vi "solar_tcp Core Server.vi"(7 "Action":T4, 8 "error in (no error)":errorcluster, 9 "Read Timeout (0ms)":i32, 10 "Message to Send":string, 11 "TCP Data in":T1 {"Debug"."Time" format="%<%Y-%m-%d\n%H:%M:%S%3u>T"}) -> (0 "error out":errorcluster, 1 "Connected":bool, 2 "Message Read/Sent":string, 3 "TCP Data out":T1 {"Debug"."Time" format="%<%Y-%m-%d\n%H:%M:%S%3u>T"})   [LabVIEW 2018]
doc: "This is the TCP Server core state machine that handles a TCP session. The <b>Message to Send</b> and <b>Message Read</b> should contain the entire TCP message including the header. Before writing the <b>Message to Send</b> the length field is updated as defined by the configuration header length offset and size. The total length field is typically the first 4 bytes of the message which includes the total packet size."
uses:
  solar_tcp_ctl Action.ctl
  solar_tcp_ctl Data.ctl
  solar_tcp_ctl Config.ctl
  solar_tcp_ctl Debug.ctl
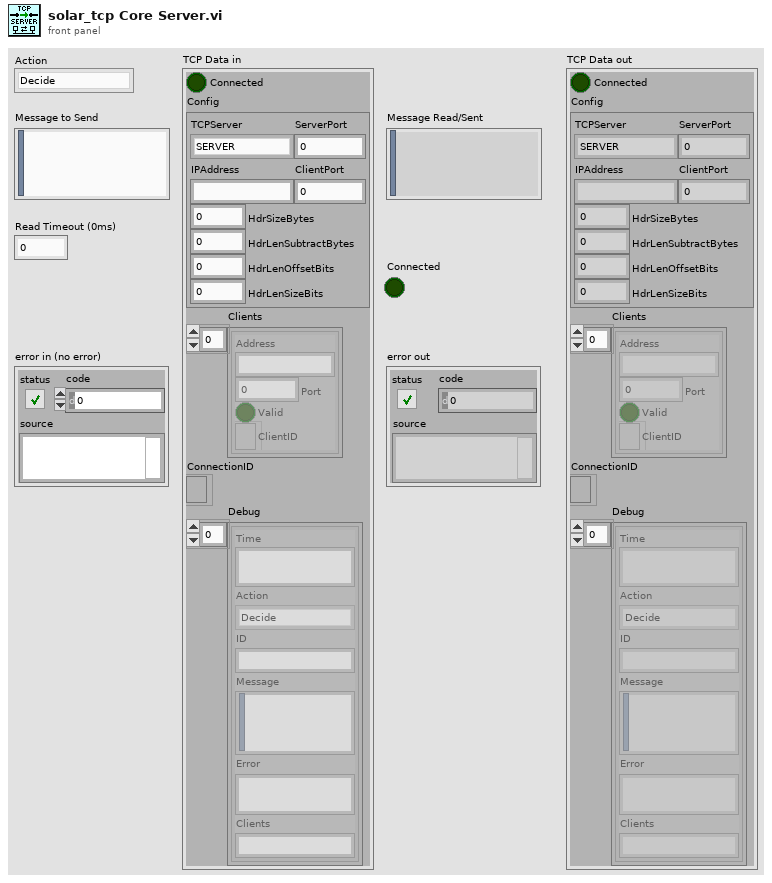
[diagram p1: front panel]
types:
  T1 = typedef "solar_tcp_ctl Data.ctl" = cluster{"Connected":bool, "Config":T2, "Clients":cluster{"Address":string, "Port":u16, "Valid":bool, "ClientID":refnum<k5>}[], "ConnectionID":refnum<k5>, "Debug":T3[]}
  T2 = typedef "solar_tcp_ctl Config.ctl" = cluster{"TCPServer":enum8{"SERVER", "CLIENT"}, "ServerPort":u16, "IPAddress":string, "ClientPort":u16, "HdrSizeBytes":i32, "HdrLenSubtractBytes":i32, "HdrLenOffsetBits":i32, "HdrLenSizeBits":i32}
  T3 = typedef "solar_tcp_ctl Debug.ctl" = cluster{"Time":timestamp, "Action":T4, "ID":string, "Message":string, "Error":string, "Clients":string}
  T4 = typedef "solar_tcp_ctl Action.ctl" = enum16{"Decide", "CreateListener", "Open", "Read", "Write", "Close", "Shutdown", "Done", "ChangePort"}
  T5 = cluster{"Address":string, "Port":u16, "Valid":bool, "ClientID":refnum<k5>}[]
  T6 = cluster{"Address":string, "Port":u16, "Valid":bool, "ClientID":refnum<k5>}
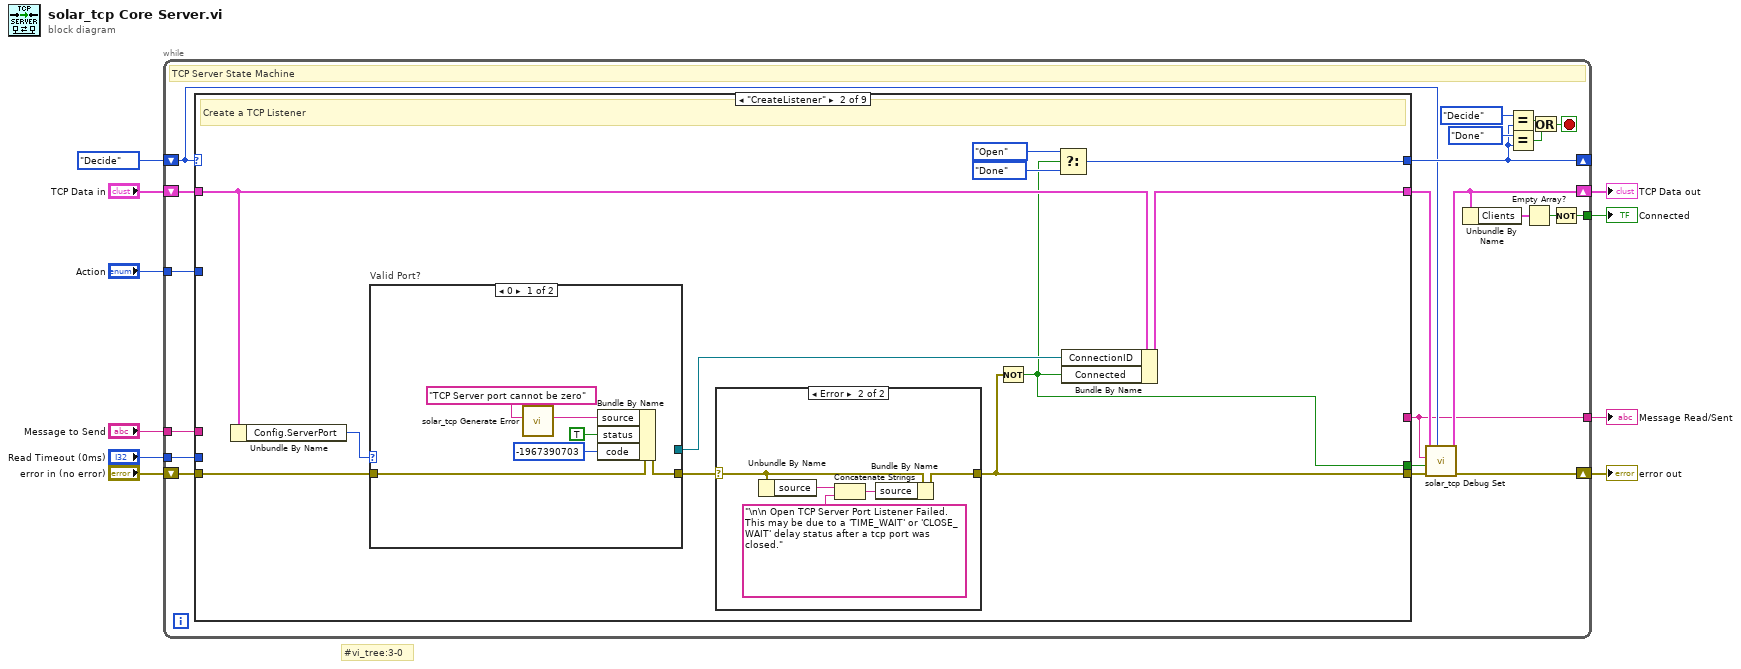
[diagram p0: block diagram]
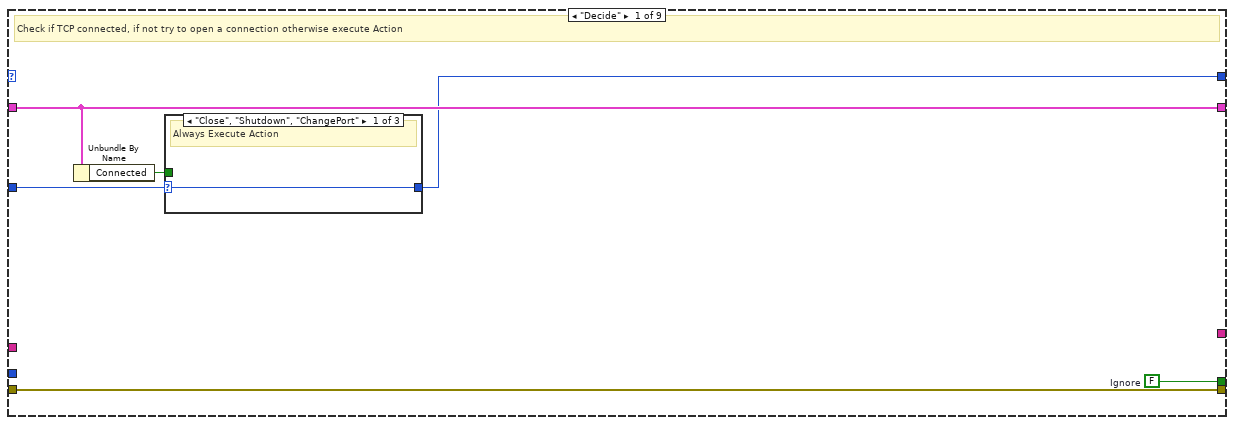
[diagram p2: hidden frame]
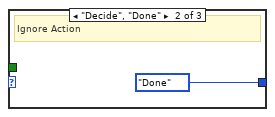
[diagram p3: hidden frame]
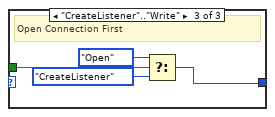
[diagram p4: hidden frame]
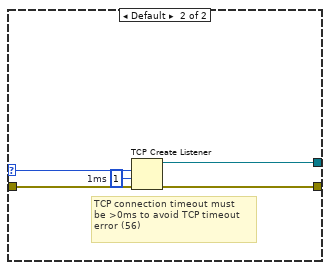
[diagram p5: hidden frame]
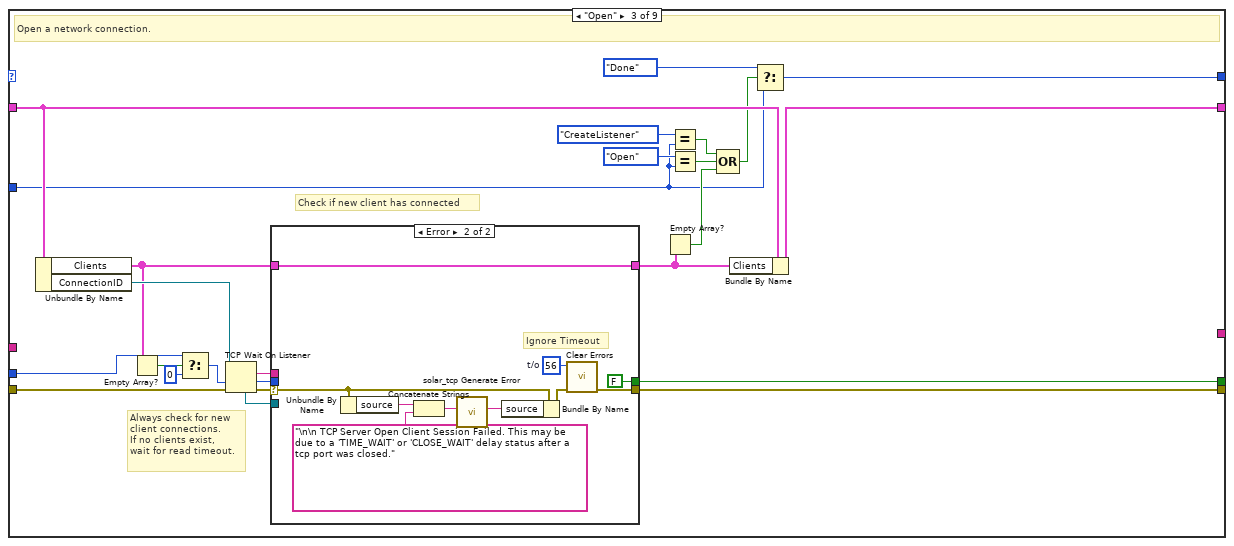
[diagram p7: hidden frame]
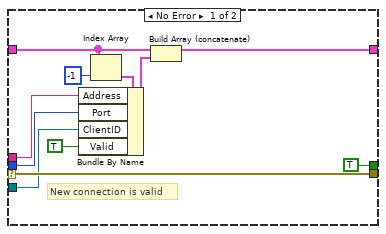
[diagram p8: hidden frame]
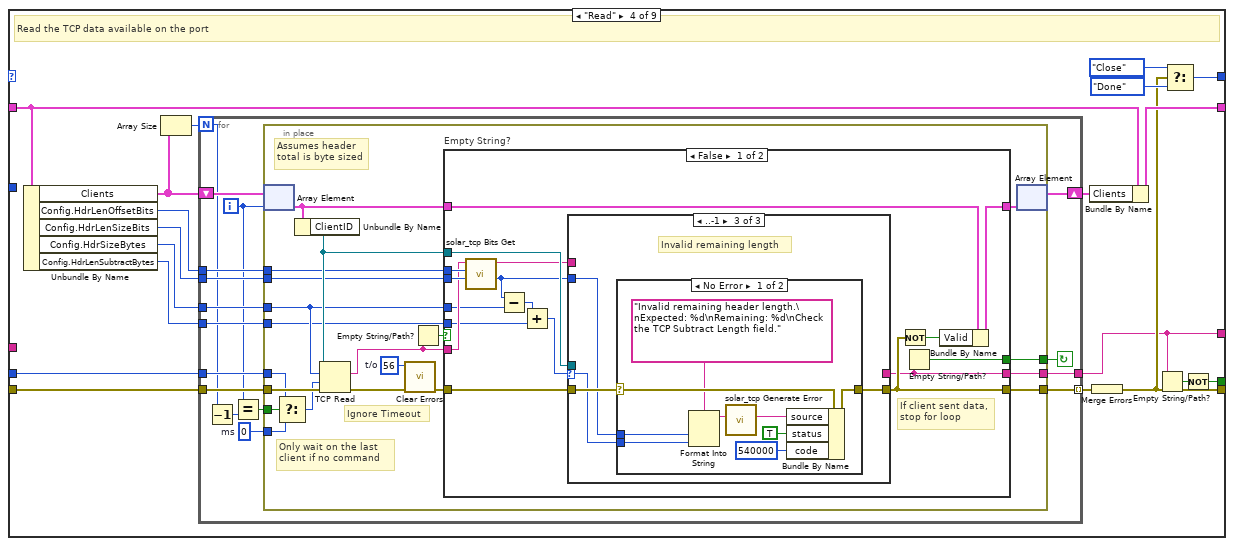
[diagram p9: hidden frame]
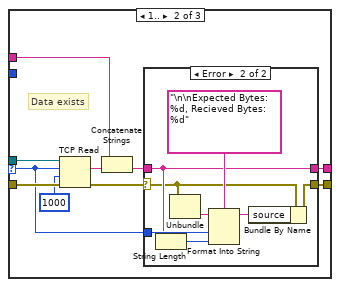
[diagram p11: hidden frame]
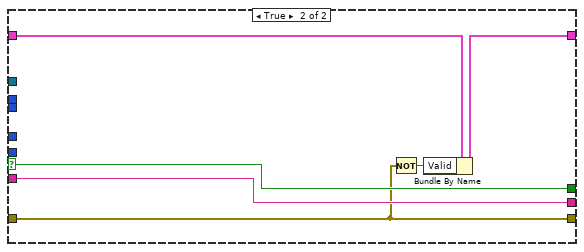
[diagram p14: hidden frame]
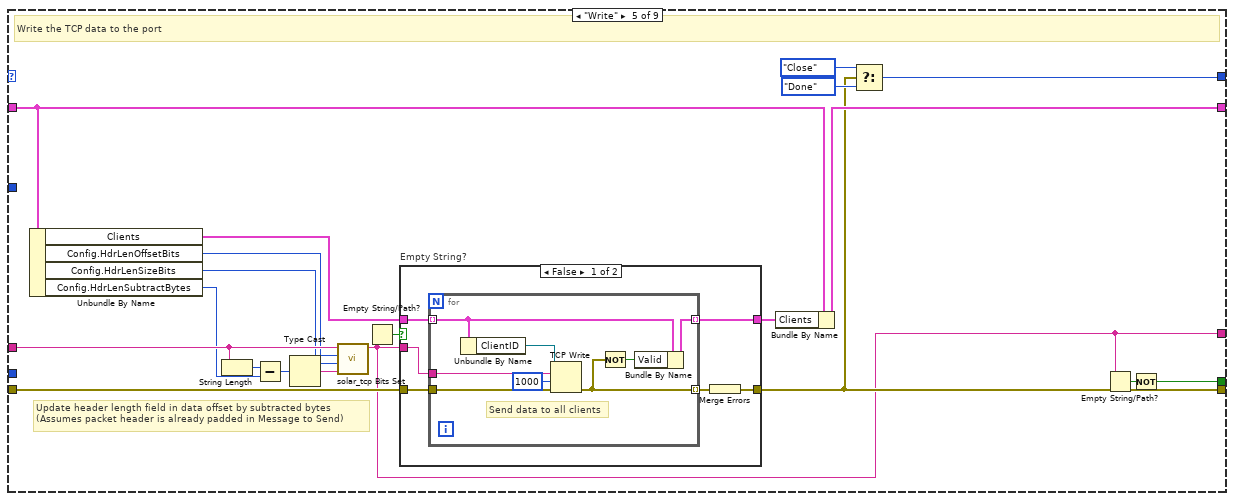
[diagram p15: hidden frame]
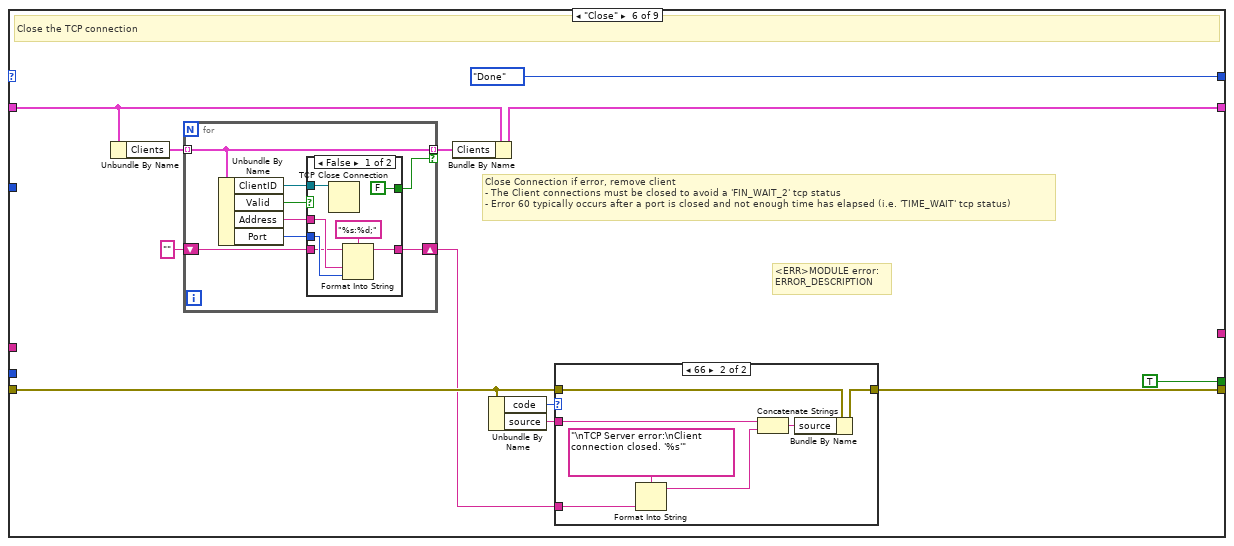
[diagram p17: hidden frame]
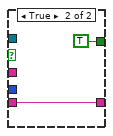
[diagram p19: hidden frame]
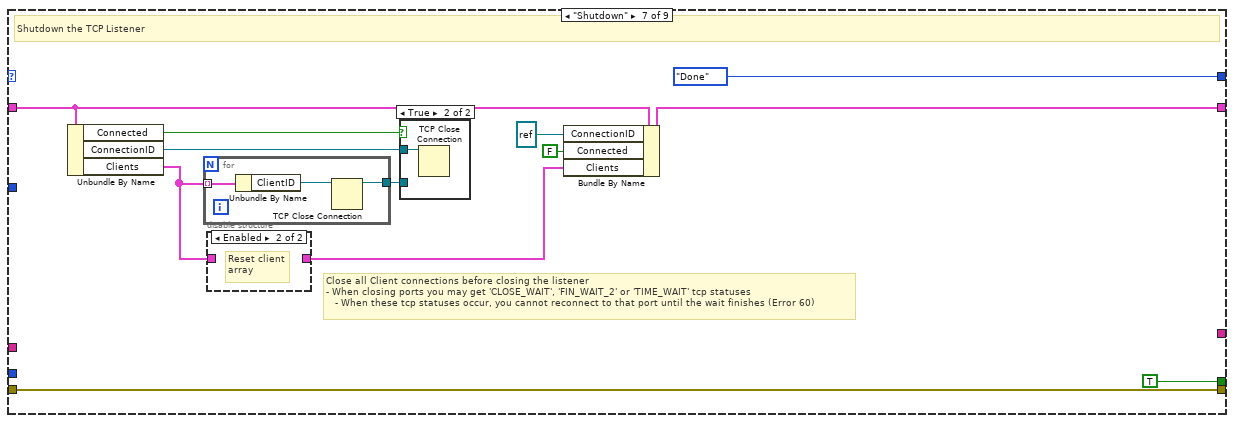
[diagram p20: hidden frame]
diagram:
  # "#vi_tree:3-0"
  n1 = while {
    shift-right: [w18] -> _
    shift-left: solar_tcp_ctl_Action."Decide" ("Function 2") -> [w13]
    shift-right: [w15] -> w5
    shift-left: "TCP Data in" -> [w31]
    tunnel: [w12] -> w10
    tunnel: "Action" -> [w25]
    tunnel: "Message to Send" -> [w24]
    shift-right: [w17] -> w1
    shift-left: "error in (no error)" -> [w23]
    tunnel: [w20] -> w4
    tunnel: "Read Timeout (0ms)" -> [w19]
    stop <- w26 stop-if-true
    # "TCP Server State Machine"
    n2 = case shown="\"CreateListener\"" w13 {
      tunnel: w31 -> [w37 w54 w96 w132 w247 w278 w315 w325 w336]
      tunnel: [w37 w53 w95 w131 w248 w277 w314 w325 w335] -> w14
      tunnel: [w35 w46 w89 w134 w249 solar_tcp_ctl_Action."Done" ("Function 2") solar_tcp_ctl_Action."Done" ("Function 2") solar_tcp_ctl_Action."Done" ("Function 2") solar_tcp_ctl_Action."CreateListener" ("Function 2")] -> w18
      tunnel: [w33 w52 w94 w129 w244 w273 w309 w323 w329] -> w16
      tunnel: [_ _ _ w120 w233 _ _ _ _] -> w12
      tunnel: w25 -> [w34 _ w73 _ _ _ _ _ _]
      tunnel: w24 -> [_ _ _ _ w238 _ _ _ _]
      tunnel: w23 -> [w33 w49 w81 w125 w243 w272 w309 w323 w329]
      tunnel: w19 -> [_ _ w78 w121 _ _ _ _ _]
      tunnel: [w32 w44 w75 w118 w232 TRUE ("Ignore") TRUE ("Ignore") FALSE ("Ignore") TRUE ("Ignore")] -> w11
      frame "Decide" {
        w32 = FALSE  # Ignore
        # "Check if TCP connected, if not try to open a connection otherwise execute Action"
        n3 = Unbundle By Name(w37) -> ("Connected"=w36:bool)
        n4 = case shown="\"Close\", \"Shutdown\", \"ChangePort\"" w34 {
          selector: w34 -> [w38 _ _]
          tunnel: w36 -> [_ _ w42]
          tunnel: [w38 solar_tcp_ctl_Action."Done" ("Function 2") w41] -> w35
          frame "Close", "Shutdown", "ChangePort" {
            # "Always Execute Action"
          }
          frame "Decide", "Done" {
            # "Ignore Action"
          }
          frame "CreateListener".."Write" {
            # "Open Connection First"
            n5 = Select(t=solar_tcp_ctl_Action."Open" ("Function 2"), s=w42, f=solar_tcp_ctl_Action."CreateListener" ("Function 2")) -> (s? t:f=w41:T4)
          }
        }
      }
      frame "CreateListener" {
        # "Create a TCP Listener"
        n6 = Unbundle By Name(w54) -> ("Config.ServerPort"=w48:u16)
        n7 = case "Valid Port?" shown="0" w48 {
          selector: w48 -> [_ w62]
          tunnel: [w60 w65] -> w51
          tunnel: [_ w64] -> w50
          tunnel: w49 -> [w55 w63]
          frame 0 {
            n8 = call "solar_tcp Generate Error.vi"("Source in"="TCP Server port cannot be zero") -> ("Source + Call Chain"=w57:string)  [unwired: 10 in]
            n9 = Bundle By Name(cluster=w55, "source"=w57, "status"=TRUE, "code"=-1967390703 ("error code (0)")) -> (w60:errorcluster)
          }
          frame Default {
            w61 = 1  # 1ms
            # "TCP connection timeout must\nbe >0ms to avoid TCP timeout\nerror (56)"
            n10 = TCP Create Listener(8:w63, 9:w61, 10:w62) -> (0:w65:errorcluster, 3:w64:refnum<k5>)  [unwired: 2 in, 1 out]
          }
        }
        n11 = case shown="Error" w51 {
          selector: w51 -> [w66 w69]
          tunnel: [w66 w68] -> w52
          frame No Error {
          }
          frame Error {
            n12 = Unbundle By Name(w69) -> ("source"=w70:string)
            n13 = Concatenate Strings(w70, "\n\n Open TCP Server Port Listener Failed. This may be due to a 'TIME_WAIT' or 'CLOSE_WAIT' delay status after a tcp port was closed.") -> (w67:string)
            n14 = Bundle By Name(cluster=w69, "source"=w67) -> (w68:errorcluster)
          }
        }
        n15 = Not(x=w52) -> (.not. x?=w44:bool)
        n16 = Select(t=solar_tcp_ctl_Action."Open" ("Action"), s=w44, f=solar_tcp_ctl_Action."Done" ("Action")) -> (s? t:f=w46:T4)
        n17 = Bundle By Name(cluster=w54, "ConnectionID"=w50, "Connected"=w44) -> (w53:T1)
      }
      frame "Open" {
        # "Always check for new\nclient connections.\nIf no clients exist,\nwait for read timeout."
        # "Check if new client has connected"
        # "Open a network connection."
        n18 = Unbundle By Name(w96) -> ("Clients"=w80:T5, "ConnectionID"=w93:refnum<k5>)
        n19 = Empty Array?(array=w80) -> (empty?=w79:bool)
        n20 = Select(t=w78, s=w79, f=0 ("ms")) -> (s? t:f=w76:i32)
        n21 = TCP Wait On Listener(8:w81, 9:w76, 11:w93) -> (0:w92:errorcluster, 1:w87:u16, 2:w86:string, 4:w88:refnum<k5>)  [unwired: 1 in, 1 out]
        n22 = case shown="Error" w92 {
          selector: w92 -> [w107 w111]
          tunnel: [w107 w114] -> w94
          tunnel: w80 -> [w101 w117]
          tunnel: [w106 w117] -> w91
          tunnel: w88 -> [w103 _]
          tunnel: w87 -> [w105 _]
          tunnel: w86 -> [w104 _]
          tunnel: [TRUE FALSE] -> w75
          frame No Error {
            # "New connection is valid"
            n23 = Index Array(array=w101, index=-1) -> (element=w99:T6)
            n24 = Bundle By Name(cluster=w99, "Address"=w104, "Port"=w105, "ClientID"=w103, "Valid"=TRUE) -> (w102:T6)
            n25 = Build Array (concatenate)(w101, w102) -> (w106:T5)
          }
          frame Error {
            w115 = 56  # t/o
            # "Ignore Timeout"
            n26 = Unbundle By Name(w111) -> ("source"=w116:string)
            n27 = Concatenate Strings(w116, "\n\n TCP Server Open Client Session Failed. This may be due to a 'TIME_WAIT' or 'CLOSE_WAIT' delay status after a tcp port was closed.") -> (w109:string)
            n28 = call "solar_tcp Generate Error.vi"("Source in"=w109) -> ("Source + Call Chain"=w108:string)  [unwired: 10 in]
            n29 = Bundle By Name(cluster=w111, "source"=w108) -> (w110:errorcluster)
            n30 = call <vilib>:"Clear Errors.vi"("error in (no error)"=w110, "specific error code to clear (0: all)"=w115) -> ("error out"=w114:errorcluster)  [unwired: 4 in, 1 out]
          }
        }
        n31 = Empty Array?(array=w91) -> (empty?=w83:bool)
        n32 = Equal?(x=solar_tcp_ctl_Action."CreateListener" ("y"), y=w73) -> (x = y?=w72:bool)
        n33 = Equal?(x=solar_tcp_ctl_Action."Open" ("y"), y=w73) -> (x = y?=w84:bool)
        n34 = Compound Arithmetic op=OR(w72, w84, w83) -> (w82:bool)
        n35 = Bundle By Name(cluster=w96, "Clients"=w91) -> (w95:T1)
        n36 = Select(t=solar_tcp_ctl_Action."Done" ("Action"), s=w82, f=w73) -> (s? t:f=w89:T4)
      }
      frame "Read" {
        # "Read the TCP data available on the port"
        n37 = Unbundle By Name(w132) -> ("Clients"=w128:T5, "Config.HdrLenOffsetBits"=w123:i32, "Config.HdrLenSizeBits"=w124:i32, "Config.HdrSizeBytes"=w133:i32, "Config.HdrLenSubtractBytes"=w122:i32)
        n38 = Array Size(array=w128) -> (size(s)=w127:i32)
        n39 = for {
          N: w127 -> [w140]
          tunnel: w133 -> [w152]
          tunnel: [w150] -> w120
          tunnel: [w151] -> w130 mode=indexing
          shift-right: [w148] -> w126
          shift-left: w128 -> [w149]
          tunnel: w125 -> [w146]
          tunnel: w124 -> [w145]
          tunnel: w123 -> [w144]
          tunnel: w122 -> [w143]
          tunnel: w121 -> [w142]
          i -> [w141]
          stop <- w147 continue-if-true
          w137 = 0  # ms
          n40 = Decrement(x=w140) -> (x-1=w139:i32)
          n41 = Equal?(x=w141, y=w139) -> (x = y?=w138:bool)
          n42 = in-place {
            in-place-border: w152 -> [w163]
            in-place-border: [w166] -> w151
            in-place-border: [w171] -> w150
            in-place-border: [w170] -> w147
            in-place-border: w146 -> [w167]
            in-place-border: w145 -> [w165]
            in-place-border: w144 -> [w164]
            in-place-border: w143 -> [w162]
            in-place-border: w142 -> [w155]
            in-place-border: w138 -> [w156]
            in-place-border: w137 -> [w154]
            w159 = 56  # t/o
            # "Only wait on the last\nclient if no command"
            # "Ignore Timeout"
            # "Assumes header \ntotal is byte sized"
            n43 = in-place-array #1(w149, w141) -> (w169:T6)
            n44 = Select(t=w155, s=w156, f=w154) -> (s? t:f=w153:i32)
            n45 = Unbundle By Name(w169) -> ("ClientID"=w172:refnum<k5>)
            n46 = TCP Read(connection ID=w172, bytes to read=w163, error in (no error)=w167, 9:w153) -> (data out=w161:string, error out=w158:errorcluster)  [unwired: 1 in, 1 out]
            n47 = call <vilib>:"Clear Errors.vi"("error in (no error)"=w158, "specific error code to clear (0: all)"=w159) -> ("error out"=w157:errorcluster)  [unwired: 4 in, 1 out]
            n48 = Empty String/Path?(string/path=w161) -> (empty?=w160:bool)
            n49 = case "Empty String?" shown="False" w160 {
              selector: w160 -> [_ w229]
              tunnel: w172 -> [w176 _]
              tunnel: [w177 w230] -> w171
              tunnel: [w189 w229] -> w170
              tunnel: w169 -> [w188 w231]
              tunnel: [w187 w228] -> w168
              tunnel: [w178 w227] -> w166
              tunnel: w157 -> [w179 w227]
              tunnel: w165 -> [w186 _]
              tunnel: w164 -> [w185 _]
              tunnel: w161 -> [w184 w230]
              tunnel: w163 -> [w183 _]
              tunnel: w162 -> [w181 _]
              frame False {
                # "If client sent data,\nstop for loop"
                n50 = call "solar_tcp Bits Get.vi"("Bit Size (0..64)"=w186, "Bit Offset (0)"=w185, "Data"=w184) -> ("Value as I32"=w173:i32, "dup Data"=w174:string)  [unwired: 6 in, 1 out]
                n51 = Subtract(x=w173, y=w183) -> (x-y=w182:i32)
                n52 = Add(x=w182, y=w181) -> (x+y=w175:i32)
                n53 = case shown="..-1" w175 {
                  selector: w175 -> [_ w195 w212]
                  tunnel: w176 -> [_ w201 _]
                  tunnel: [w190 w200 w214] -> w178
                  tunnel: [w191 w199 _] -> w177
                  tunnel: w179 -> [w190 w198 w215]
                  tunnel: w174 -> [w191 w192 _]
                  tunnel: w173 -> [_ _ w213]
                  frame 0 {
                    # "No more data expected\n- Return tcp data"
                  }
                  frame 1.. {
                    # "Data exists"
                    n54 = TCP Read(connection ID=w201, bytes to read=w195, error in (no error)=w198, 9:1000 ("Timeout (ms)")) -> (data out=w196:string, error out=w197:errorcluster)  [unwired: 1 in, 1 out]
                    n55 = Concatenate Strings(w192, w196) -> (w193:string)
                    n56 = case shown="Error" w197 {
                      selector: w197 -> [w203 w205]
                      tunnel: w193 -> [w202 w206]
                      tunnel: w195 -> [_ w209]
                      tunnel: [w203 w208] -> w200
                      tunnel: [w202 w206] -> w199
                      frame No Error {
                        # "Return entire message\n(including header)"
                      }
                      frame Error {
                        n57 = String Length(string=w206) -> (length=w211:i32)
                        n58 = Unbundle(w205) -> ("source"=w204:string)  [unwired: 2 out]
                        n59 = Format Into String(format string="\n\nExpected Bytes: %d, Recieved Bytes: %d" ("source"), initial string=w204, w209, w211) -> (resulting string=w207:string)  [unwired: 1 in, 1 out]
                        n60 = Bundle By Name(cluster=w205, "source"=w207) -> (w208:errorcluster)
                      }
                    }
                  }
                  frame ..-1 {
                    # "Invalid remaining length"
                    n61 = case shown="No Error" w215 {
                      selector: w215 -> [w224 w225]
                      tunnel: [w223 w225] -> w214
                      tunnel: w213 -> [w219 _]
                      tunnel: w212 -> [w218 _]
                      frame No Error {
                        n62 = Format Into String(format string="Invalid remaining header length.\nExpected: %d\nRemaining: %d\nCheck the TCP Subtract Length field.", w219, w218) -> (resulting string=w216:string)  [unwired: 2 in, 1 out]
                        n63 = call "solar_tcp Generate Error.vi"("Source in"=w216) -> ("Source + Call Chain"=w217:string)  [unwired: 10 in]
                        n64 = Bundle By Name(cluster=w224, "source"=w217, "status"=TRUE, "code"=540000 ("Code (540000)")) -> (w223:errorcluster)
                      }
                      frame Error {
                      }
                    }
                  }
                }
                n65 = Not(x=w178) -> (.not. x?=w180:bool)
                n66 = Empty String/Path?(string/path=w177) -> (empty?=w189:bool)
                n67 = Bundle By Name(cluster=w188, "Valid"=w180) -> (w187:T6)
              }
              frame True {
                n68 = Not(x=w227) -> (.not. x?=w226:bool)
                n69 = Bundle By Name(cluster=w231, "Valid"=w226) -> (w228:T6)
              }
            }
            n70 = in-place-array #1(w168) -> (w148:T5)  [unwired: 1 out]
          }
        }
        n71 = Bundle By Name(cluster=w132, "Clients"=w126) -> (w131:T1)
        n72 = Merge Errors(w130) -> (w129:errorcluster)
        n73 = Empty String/Path?(string/path=w120) -> (empty?=w119:bool)
        n74 = Select(t=solar_tcp_ctl_Action."Close" ("Function 2"), s=w129, f=solar_tcp_ctl_Action."Done" ("Function 2")) -> (s? t:f=w134:T4)
        n75 = Not(x=w119) -> (.not. x?=w118:bool)
      }
      frame "Write" {
        # "Update header length field in data offset by subtracted bytes\n(Assumes packet header is already padded in Message to Send)"
        # "Write the TCP data to the port"
        n76 = Unbundle By Name(w247) -> ("Clients"=w246:T5, "Config.HdrLenOffsetBits"=w235:i32, "Config.HdrLenSizeBits"=w236:i32, "Config.HdrLenSubtractBytes"=w237:i32)
        n77 = String Length(string=w238) -> (length=w241:i32)
        n78 = Subtract(x=w241, y=w237) -> (x-y=w240:i32)
        n79 = Type Cast(x=w240) -> (*(type *) &x=w239:string)  [unwired: 1 in]
        n80 = call "solar_tcp Bits Set.vi"("Value (Binary) [Byte Aligned]"=w239, "Bit Size (0..64)"=w236, "Bit Offset (0)"=w235, "Buffered Data in"=w238) -> ("Data out"=w233:string)  [unwired: 7 in]
        n81 = Empty String/Path?(string/path=w233) -> (empty?=w242:bool)
        n82 = case "Empty String?" shown="False" w242 {
          tunnel: w246 -> [w256 w267]
          tunnel: [w255 w267] -> w245
          tunnel: [w254 w266] -> w244
          tunnel: w243 -> [w253 w266]
          tunnel: w233 -> [w252 _]
          frame False {
            n83 = for {
              tunnel: w252 -> [w264]
              tunnel: [w259] -> w257 mode=indexing
              tunnel: w256 -> [w262] mode=indexing
              tunnel: [w261] -> w255 mode=indexing
              tunnel: w253 -> [w260]
              # "Send data to all clients"
              n84 = Unbundle By Name(w262) -> ("ClientID"=w263:refnum<k5>)
              n85 = TCP Write(connection ID=w263, data in=w264, error in (no error)=w260, 9:1000 ("timeout ms (25000)")) -> (error out=w259:errorcluster)  [unwired: 2 out]
              n86 = Not(x=w259) -> (.not. x?=w258:bool)
              n87 = Bundle By Name(cluster=w262, "Valid"=w258) -> (w261:T6)
            }
            n88 = Merge Errors(w257) -> (w254:errorcluster)
          }
          frame True {
          }
        }
        n89 = Bundle By Name(cluster=w247, "Clients"=w245) -> (w248:T1)
        n90 = Select(t=solar_tcp_ctl_Action."Close" ("Function 2"), s=w244, f=solar_tcp_ctl_Action."Done" ("Function 2")) -> (s? t:f=w249:T4)
        n91 = Empty String/Path?(string/path=w233) -> (empty?=w234:bool)
        n92 = Not(x=w234) -> (.not. x?=w232:bool)
      }
      frame "Close" {
        # "<ERR>MODULE error:\nERROR_DESCRIPTION"
        # "Close Connection if error, remove client\n- The Client connections must be closed to avoid a 'FIN_WAIT_2' tcp status\n- Error 60 typically occurs after a port is closed and not enough time has elapsed (i.e. 'TIME_WAIT' tcp status)"
        # "Close the TCP connection"
        n93 = Unbundle By Name(w278) -> ("Clients"=w276:T5)
        n94 = for {
          tunnel: w276 -> [w293] mode=indexing
          tunnel: [w293] -> w275 mode=indexing if=w292
          shift-right: [w289] -> w268
          shift-left: "" -> [w288]
          n95 = Unbundle By Name(w293) -> ("ClientID"=w294:refnum<k5>, "Valid"=w295:bool, "Address"=w291:string, "Port"=w290:u16)
          n96 = case shown="False" w295 {
            tunnel: w294 -> [w302 _]
            tunnel: [FALSE TRUE] -> w292
            tunnel: w291 -> [w299 _]
            tunnel: w290 -> [w298 _]
            tunnel: [w297 w303] -> w289
            tunnel: w288 -> [w296 w303]
            frame False {
              n97 = TCP Close Connection(connection ID=w302) -> ()  [unwired: 2 in, 2 out]
              n98 = Format Into String(format string="%s:%d;", initial string=w296, w299, w298) -> (resulting string=w297:string)  [unwired: 1 in, 1 out]
            }
            frame True {
            }
          }
        }
        n99 = Bundle By Name(cluster=w278, "Clients"=w275) -> (w277:T1)
        n100 = Unbundle By Name(w272) -> ("code"=w271:i32, "source"=w270:string)
        n101 = case shown="66" w271 {
          tunnel: [w280 w286] -> w273
          tunnel: w272 -> [w280 w287]
          tunnel: w270 -> [_ w285]
          tunnel: w268 -> [_ w281]
          frame Default {
          }
          frame 66 {
            n102 = Format Into String(format string="\nTCP Server error:\nClient connection closed. '%s'", w281) -> (resulting string=w282:string)  [unwired: 2 in, 1 out]
            n103 = Concatenate Strings(w285, w282) -> (w284:string)
            n104 = Bundle By Name(cluster=w287, "source"=w284) -> (w286:errorcluster)
          }
        }
      }
      frame "Shutdown" {
        # "Close all Client connections before closing the listener\n- When closing ports you may get 'CLOSE_WAIT', 'FIN_WAIT_2' or 'TIME_WAIT' tcp statuses\n   - When these tcp statuses occur, you cannot reconnect to that port until the wait finishes (Error 60)"
        # "Shutdown the TCP Listener"
        n105 = Unbundle By Name(w315) -> ("Connected"=w311:bool, "ConnectionID"=w310:refnum<k5>, "Clients"=w307:T5)
        n106 = for {
          tunnel: w307 -> [w320] mode=indexing
          tunnel: [w318] -> w306
          n107 = Unbundle By Name(w320) -> ("ClientID"=w319:refnum<k5>)
          n108 = TCP Close Connection(connection ID=w319) -> (connection ID out=w318:refnum<k5>)  [unwired: 2 in, 1 out]
        }
        n109 = disable-structure shown="Enabled" {
          disable-tunnel: [w317 _] -> w308
          disable-tunnel: w307 -> [w317 _]
          frame Disabled {
          }
          frame Enabled {
            # "Reset client\narray"
          }
        }
        n110 = case shown="True" w311 {
          tunnel: w310 -> [_ w321]
          tunnel: w306 -> [_ _]
          frame False {
          }
          frame True {
            n111 = TCP Close Connection(connection ID=w321) -> ()  [unwired: 2 in, 2 out]
          }
        }
        n112 = Bundle By Name(cluster=w315, "ConnectionID"=refnum<k5> refnum ("Connection ID"), "Connected"=FALSE, "Clients"=w308) -> (w314:T1)
      }
      frame "Done" {
        # "Do Nothing"
      }
      frame "ChangePort" {
        # "Close the TCP connection and try to reopen the connection"
        n113 = Unbundle By Name(w336) -> ("Connected"=w332:bool, "ConnectionID"=w331:refnum<k5>, "Clients"=w328:T5)
        n114 = for {
          tunnel: w328 -> [w341] mode=indexing
          tunnel: [w339] -> w330
          n115 = Unbundle By Name(w341) -> ("ClientID"=w340:refnum<k5>)
          n116 = TCP Close Connection(connection ID=w340) -> (connection ID out=w339:refnum<k5>)  [unwired: 2 in, 1 out]
        }
        n117 = disable-structure shown="Enabled" {
          disable-tunnel: [w338 _] -> w327
          disable-tunnel: w328 -> [w338 _]
          frame Disabled {
          }
          frame Enabled {
            # "Reset client\narray"
          }
        }
        n118 = case shown="True" w332 {
          tunnel: w331 -> [_ w342]
          tunnel: w330 -> [_ _]
          frame False {
          }
          frame True {
            n119 = TCP Close Connection(connection ID=w342) -> ()  [unwired: 2 in, 2 out]
          }
        }
        n120 = Bundle By Name(cluster=w336, "ConnectionID"=refnum<k5> refnum ("Connection ID"), "Connected"=FALSE, "Clients"=w327) -> (w335:T1)
      }
    }
    n121 = call "solar_tcp Debug Set.vi"("Action"=w13, "error in (no error)"=w16, "Update? (T)"=w11, "Message Sent/Read"=w12, "TCP Data in"=w14) -> ("error out"=w17:errorcluster, "TCP Data out"=w15:T1)  [unwired: 5 in]
    n122 = Unbundle By Name(w15) -> ("Clients"=w22:T5)
    n123 = Equal?(x=solar_tcp_ctl_Action."Decide" ("Function 2"), y=w18) -> (x = y?=w28:bool)
    n124 = Equal?(x=solar_tcp_ctl_Action."Done" ("Function 2"), y=w18) -> (x = y?=w27:bool)
    n125 = Empty Array?(array=w22) -> (empty?=w21:bool)
    n126 = Or(x=w28, y=w27) -> (x .or. y?=w26:bool)
    n127 = Not(x=w21) -> (.not. x?=w20:bool)
  }
  "error out" <- w1
  "Message Read/Sent" <- w10
  "TCP Data out" <- w5
  "Connected" <- w4
